vi "ED3.vi"() -> ()   [LabVIEW 2015]
uses:
  <vilib>/Instr/_visa.llb/VISA Flush IO Buffer Mask.ctl
  <vilib>/Instr/_visa.llb/VISA Configure Serial Port (Instr).vi
panel:
  in  "Cluster":T1
  out "Planta_out":sgl(graph)
  in  "Boolean":bool
  out "Planta_in":sgl(graph)
  out "Error":sgl(graph)
  out "Channel 1":u16(graph)
  out "Cluster 3":T2
  in  "Serial Settings 2":T3={"baud rate"=9600, "data bits"=8, "parity"=enum."None", "stop bits"=10, "flow control"=0} {"flow control" items=["None"=0, "XON/XOFF"=1, "RTS/CTS"=2, "DTR/DSR"=4]; "stop bits" items=["1.0"=10, "1.5"=15, "2.0"=20]; "data bits" min=5 max=8 step=1; "baud rate" items=["75"=75, "110"=110, "134"=134, "150"=150, "300"=300, "600"=600, "1200"=1200, "1800"=1800, "2400"=2400, "4800"=4800, "7200"=7200, "9600"=9600, "14400"=14400, "19200"=19200, "28800"=28800, "38400"=38400, "56000"=56000, "57600"=57600, "115200"=115200, "128000"=128000, "230400"=230400]}
  in  "EDU-CIAA":refnum<visa-resource-name>
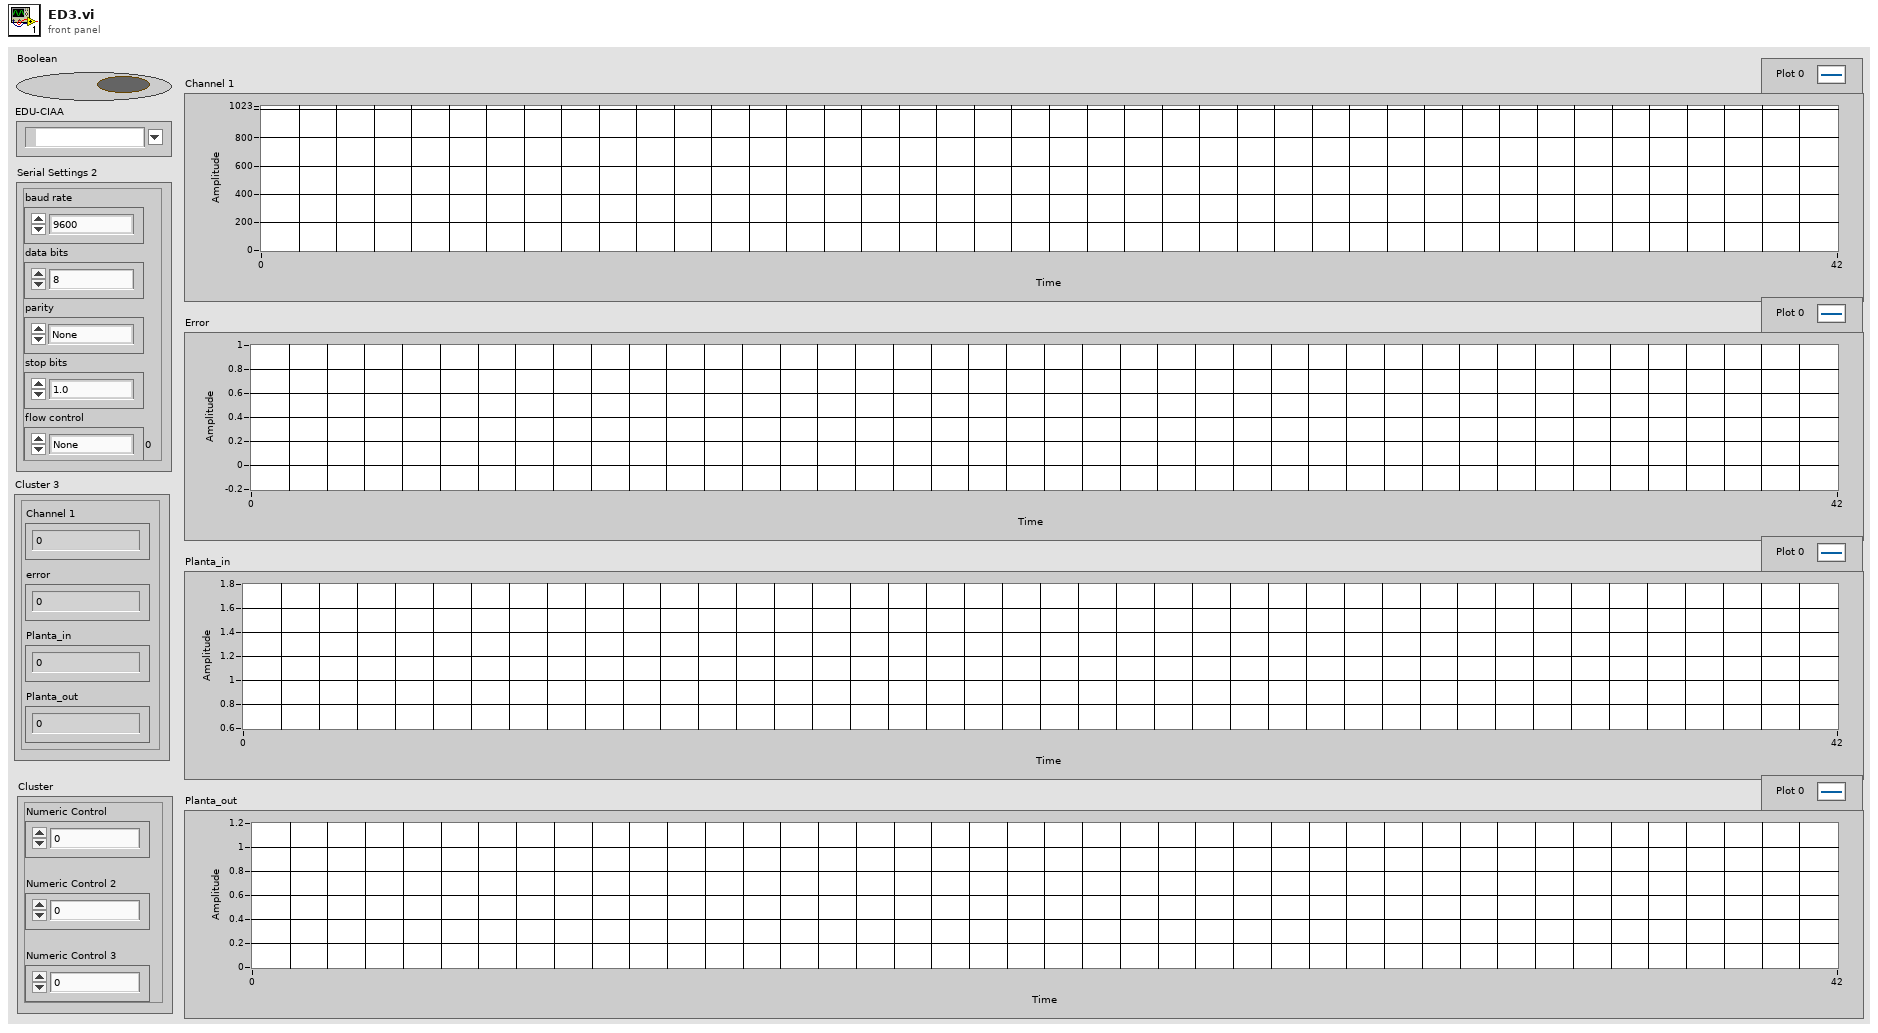
[diagram p1: front panel]
types:
  T1 = cluster{"Numeric Control":sgl, "Numeric Control 2":sgl, "Numeric Control 3":sgl}
  T2 = cluster{"Channel 1":u16, "error":sgl, "Planta_in":sgl, "Planta_out":sgl}
  T3 = cluster{"baud rate":u32, "data bits":u16, "parity":enum16{"None", "Odd", "Even", "Mark", "Space"}, "stop bits":u16, "flow control":u16}
  T4 = typedef "VISA Flush IO Buffer Mask.ctl" = u16
  T5 = enum16{"big-endian, network order", "native, host order", "little-endian"}
  T6 = cluster{"Numeric Control":u16, "Numeric Control 2":sgl, "Numeric Control 3":sgl, "Numeric Control 4":sgl}
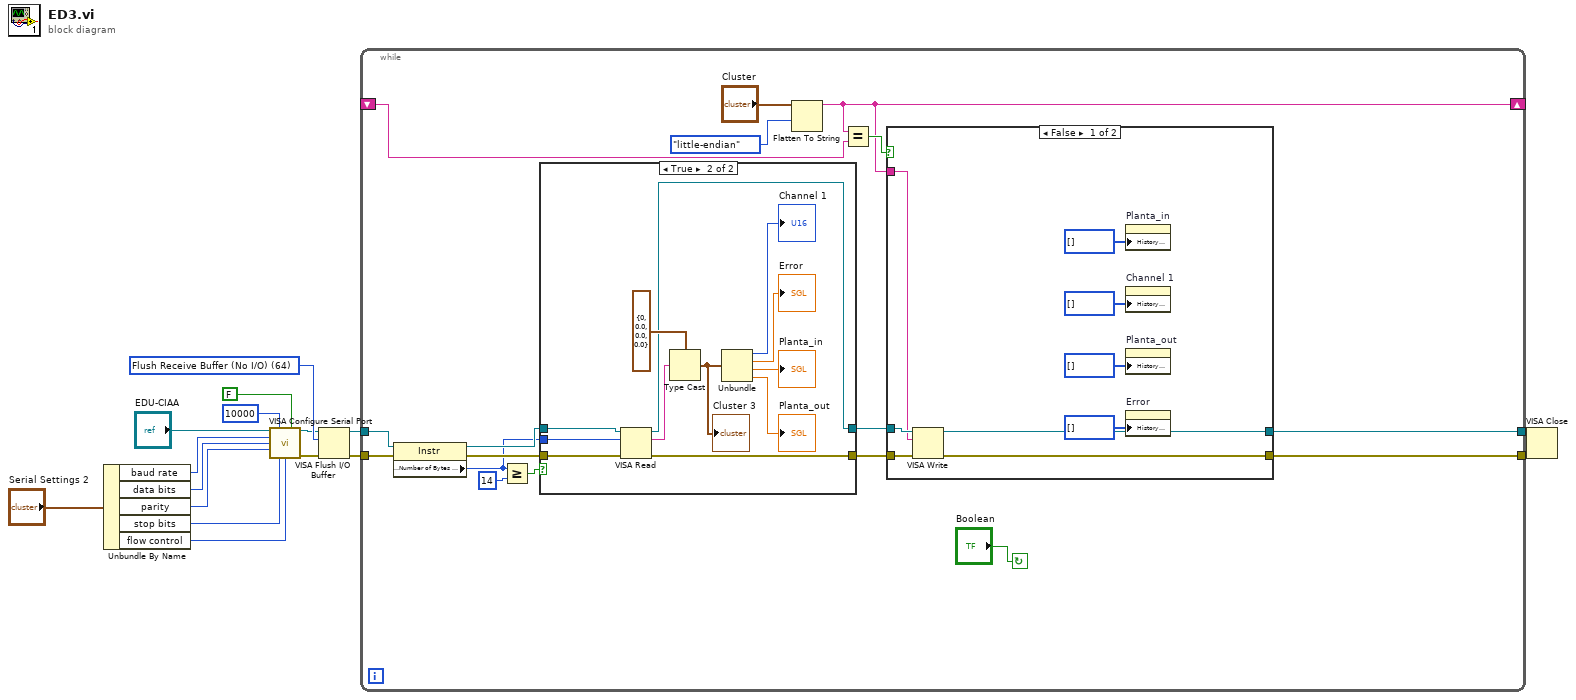
[diagram p0: block diagram]
diagram:
  w8 = T4 64 items=["Flush Receive Buffer"=16, "Write Transmit Buffer to Device"=32, "Flush Receive Buffer (No I/O)"=64, "Flush Transmit Buffer"=128] ("Mask")
  n1 = Unbundle By Name("Serial Settings 2") -> ("baud rate"=w14:u32, "data bits"=w13:u16, "parity"=w12:enum16{"None", "Odd", "Even", "Mark", "Space"}, "stop bits"=w11:u16, "flow control"=w10:u16)
  n2 = call-poly "VISA Configure Serial Port"("VISA resource name"="EDU-CIAA", "timeout (10sec)"=u32 10000, "Enable Termination\nChar (T)"=FALSE ("Enable Termination\nChar (T)"), "baud rate (9600)"=w14, "data bits (8)"=w13, "parity (0:none)"=w12, "stop bits (10: 1 bit)"=w11, "flow control (0:none)"=w10) -> ("VISA resource name out"=w2:refnum<visa-resource-name>, "error out"=w1:errorcluster)  [unwired: 6 in]
  n3 = VISA Flush I/O Buffer(VISA resource name=w2, mask (16)=w8, error in (no error)=w1) -> (VISA resource name out=w4:refnum<visa-resource-name>, error out=w3:errorcluster)
  n4 = while {
    tunnel: w4 -> [w26]
    tunnel: w3 -> [w25]
    tunnel: [w30] -> w7
    tunnel: [w29] -> w6
    shift-right: [w19] -> _
    shift-left: _ -> [w27]
    stop <- "Boolean" continue-if-true
    n5 = property class="Instr"(reference=w26, error in=w25) -> (reference out=w24:refnum<visa-resource-name>, error out=w23:errorcluster, "Serial Settings:Number of Bytes at Serial Port"=w17:u32)
    n6 = Greater Or Equal?(x=w17, y=u32 14) -> (x >= y?=w21:bool)
    n7 = case shown="True" w21 {
      tunnel: [w46 w53] -> w32
      tunnel: [w45 w52] -> w31
      tunnel: w23 -> [w45 w51]
      tunnel: w24 -> [w46 w50]
      tunnel: w17 -> [_ w47]
      frame False {
      }
      frame True {
        n8 = VISA Read(VISA resource name=w50, byte count=w47, error in (no error)=w51) -> (VISA resource name out=w53:refnum<visa-resource-name>, read buffer=w57:string, error out=w52:errorcluster)  [unwired: 1 out]
        n9 = Type Cast(type=T6 {"Numeric Control"=0, "Numeric Control 2"=0.0, "Numeric Control 3"=0.0, "Numeric Control 4"=0.0} ("Cluster"), x=w57) -> (*(type *) &x=w49:T6)
        "Cluster 3" <- w49
        n10 = Unbundle(w49) -> ("Numeric Control"=→"Channel 1":u16, "Numeric Control 2"=→"Error":sgl, "Numeric Control 3"=→"Planta_in":sgl, "Numeric Control 4"=→"Planta_out":sgl)
      }
    }
    n11 = Flatten To String(anything="Cluster", byte order (0:big-endian, network order)=T5."little-endian") -> (data string=w19:string)  [unwired: 2 in, 2 out]
    n12 = Equal?(x=w19, y=w27) -> (x = y?=w28:bool)
    n13 = case shown="False" w28 {
      tunnel: w32 -> [w42 w44]
      tunnel: w31 -> [w39 w43]
      tunnel: [w41 w44] -> w30
      tunnel: [w38 w43] -> w29
      tunnel: w19 -> [w40 _]
      frame False {
        n14 = VISA Write(VISA resource name=w42, write buffer=w40, error in (no error)=w39) -> (VISA resource name out=w41:refnum<visa-resource-name>, error out=w38:errorcluster)  [unwired: 1 out]
        n15 = property on="Planta_in" class="WFChart (strict)"("History Data"=i32[] []) -> ()  [unwired: 2 in, 2 out]
        n16 = property on="Channel 1" class="WFChart (strict)"("History Data"=u16[] []) -> ()  [unwired: 2 in, 2 out]
        n17 = property on="Planta_out" class="WFChart (strict)"("History Data"=i32[] []) -> ()  [unwired: 2 in, 2 out]
        n18 = property on="Error" class="WFChart (strict)"("History Data"=i32[] []) -> ()  [unwired: 2 in, 2 out]
      }
      frame True {
      }
    }
  }
  n19 = VISA Close(VISA resource name=w7, error in (no error)=w6) -> ()  [unwired: 1 out]
